vi "4.6.3.vi"() -> ()   [LabVIEW 2017]
panel:
  in  "停止":bool
  in  "B":dbl
  out "和":dbl
  in  "A":dbl
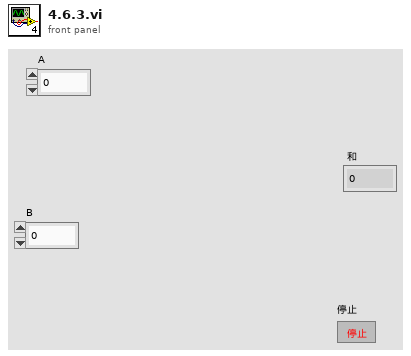
[diagram p1: front panel]
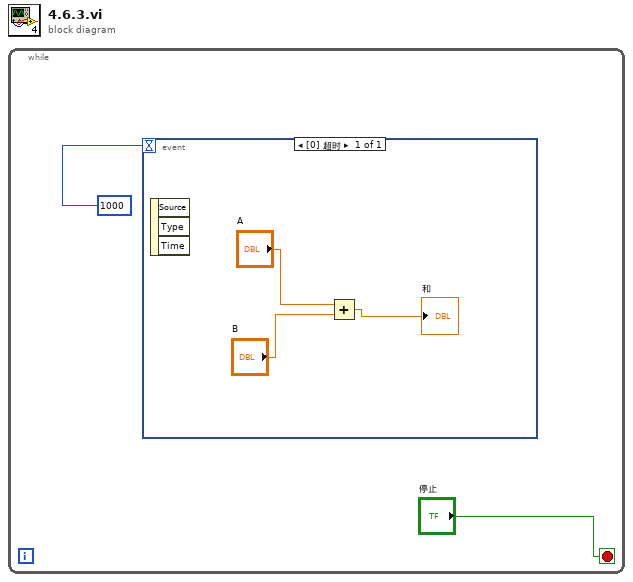
[diagram p0: block diagram]
diagram:
  n1 = while {
    stop <- "停止" stop-if-true
    n2 = event shown="[0] 超时" {
      selector: _ -> [_]
      dyn-events: _ -> [_]
      timeout: 1000 -> [_]
      event Timeout {
        n3 = event-data() -> ()  [unwired: 1 in, 3 out]
        n4 = Add(x="A", y="B") -> (x+y=→"和":dbl)
      }
    }
  }
